vi "Create Resources.vi"(10 "m_axis_tdata":refnum<k21>, 11 "m_axis_tvalid":refnum<k21>) -> (3 "niInstr AXI4-Stream Reader FXP64x1 v1 FPGA out":refnum<class "niInstr AXI4-Stream Reader FXP64x1 v1 FPGA.lvclass">)   [LabVIEW 2015, in "niInstr AXI4-Stream Reader FXP64x1 v1 FPGA.lvclass"]
doc: "Creates a new FPGA resource of the selected type.\n\n<b>Do not place this VI into a case structure or it will not compile correctly!</b>\n\n<B>Input Parameters</B>\n\n<B>m_axis_tdata</B> is the resource to use as TDATA.\n\n<B>m_axis_tvalid</B> is the resource to use as TVALID.\n\n<B>Output Parameters</B>\n\n<B>niInstr AXI4-Stream Reader FXP64x1 v1 FPGA out</B> passes a reference to the AXI4-Stream Reader to the next VI."
uses:
  <instrlib>/_niInstr/CLIP Adapters/v1/FPGA/AXI4-Stream/Reader FXP64x1/niInstr AXI4-Stream Reader FXP64x1 v1 FPGA.lvclass
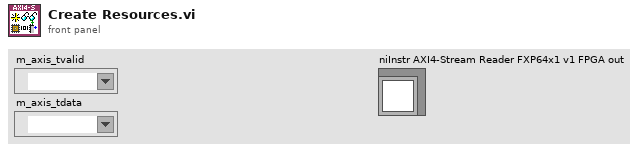
[diagram p1: front panel]
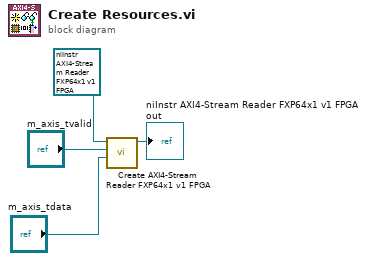
[diagram p0: block diagram]
diagram:
  n1 = call <instrlib>:"Create AXI4-Stream Reader FXP64x1 v1 FPGA.vi"("tdata"="m_axis_tdata", "tvalid"="m_axis_tvalid", "niInstr AXI4-Stream Reader FXP64x1 v1 FPGA in"=refnum<class "niInstr AXI4-Stream Reader FXP64x1 v1 FPGA.lvclass"> refnum ("Reader in")) -> ("niInstr AXI4-Stream Reader FXP64x1 v1 FPGA out"=→"niInstr AXI4-Stream Reader FXP64x1 v1 FPGA out":refnum<class "niInstr AXI4-Stream Reader FXP64x1 v1 FPGA.lvclass">)  [unwired: 8 in]
